vi "RT Main_V1 bis.vi"   [LabVIEW 2015]
doc: "This template is for the Queued Message Handler design pattern.\n\nThe Event Handling Loop generates messages based on user interface actions.\n\nThe Message Handling Loop processes messages generated by the Event Handling Loop, or by other messages. The messages are string values, so new messages can be added easily to the Message Cases case structure in the Message Handling Loop. Each message cluster can also provide an optional value for Message Data, which is a variant that can be converted to whatever message-specific data is required."
uses:
  support/Message Queue/Message Queue.lvlib
  Globals/Global - All RT Loop Stop.vi
  Globals/Global - Configuration Options.vi
  Globals/Global - RT Stream Connections.vi
  Globals/Global - Monitoring Variables.vi
  <vilib>/nisyscfg/nisyscfg.lvlib
types:
  T1 = typedef "Message Queue.lvlib/All Real-Time Message Queues.ctl" = cluster{"Message Handler":refnum<queue>, "Acquisition and Logging":refnum<queue>}
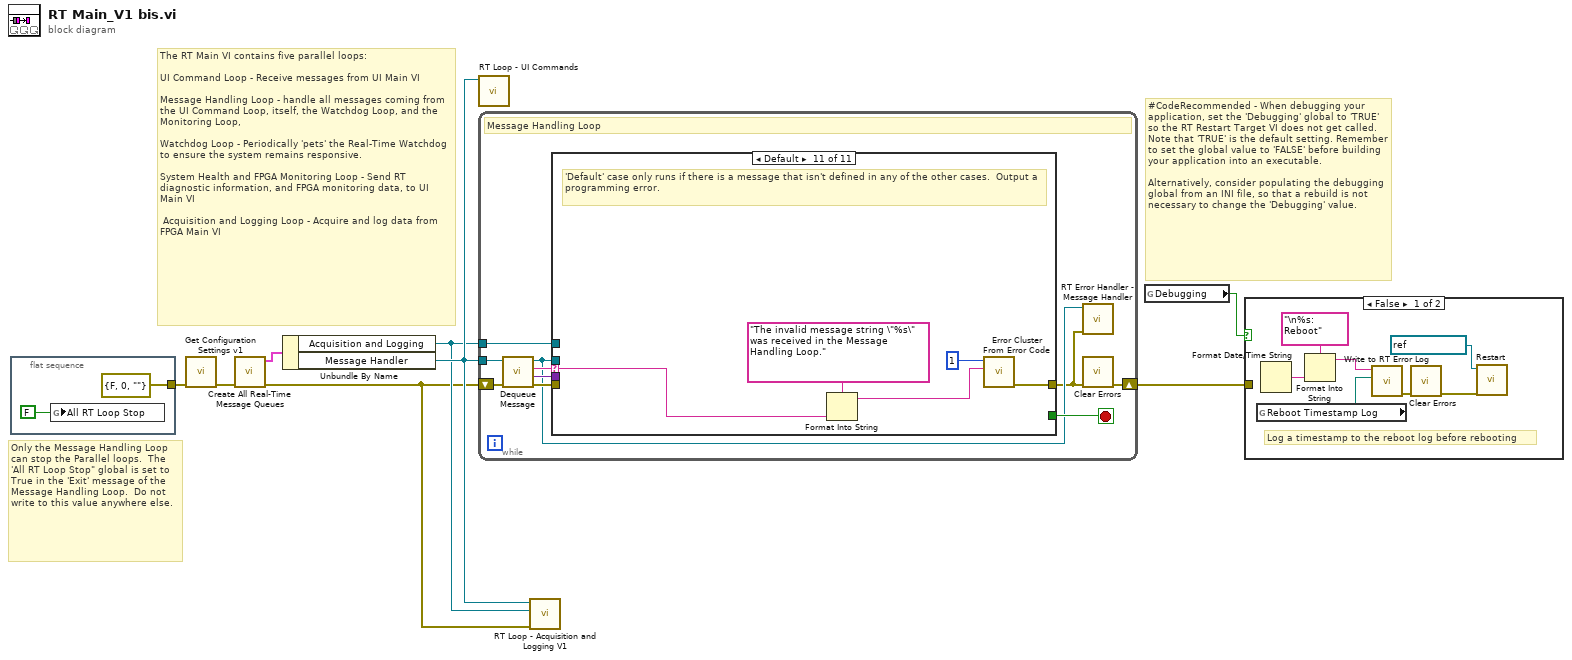
[diagram p0: block diagram]
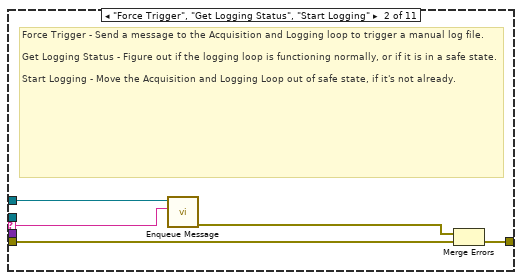
[diagram p4: hidden frame]
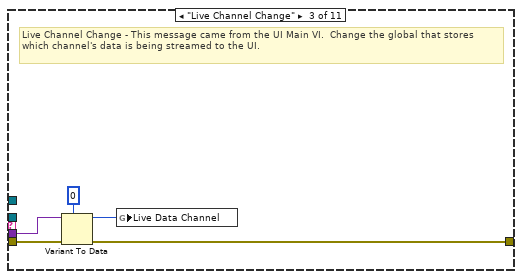
[diagram p5: hidden frame]
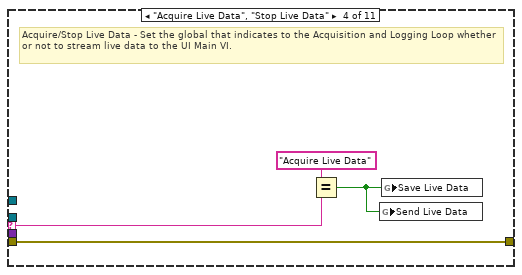
[diagram p6: hidden frame]
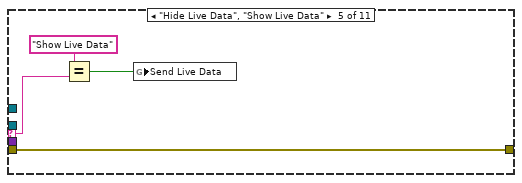
[diagram p7: hidden frame]
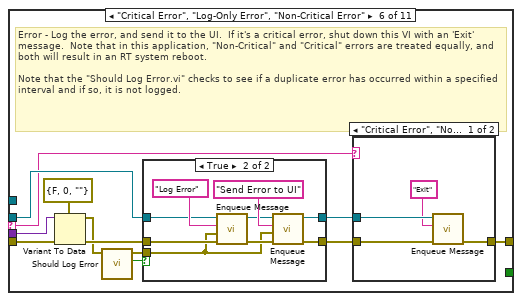
[diagram p8: hidden frame]
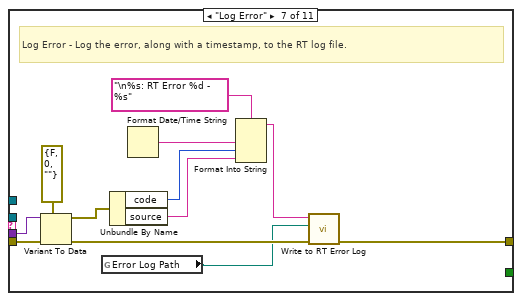
[diagram p11: hidden frame]
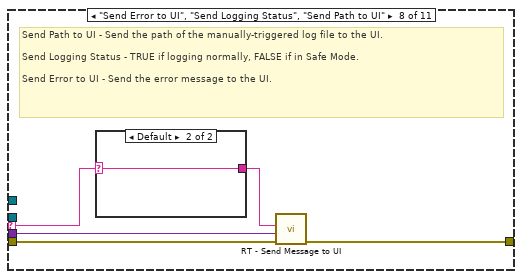
[diagram p12: hidden frame]
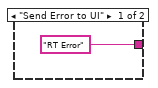
[diagram p13: hidden frame]
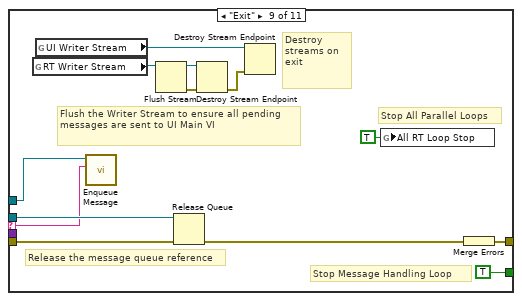
[diagram p14: hidden frame]
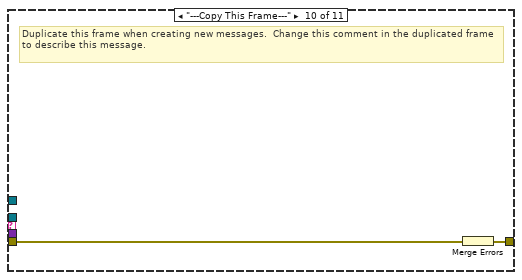
[diagram p15: hidden frame]
diagram:
  # "#CodeRecommended - When debugging your application, set the 'Debugging' global to 'TRUE' so the RT Restart Target VI does not get called.  Note that 'TRUE' is the default setting. Remember to set the global value to 'FALSE' before building your application into an executable.\n\nAlternatively, consider populating the debugging global from an INI file, so that a rebuild is not necessary to change the 'Debugging' value."
  # "The RT Main VI contains five parallel loops:\n\nUI Command Loop - Receive messages from UI Main VI\n\nMessage Handling Loop - handle all messages coming from the UI Command Loop, itself, the Watchdog Loop, and the Monitoring Loop, \n\nWatchdog Loop - Periodically 'pets' the Real-Time Watchdog to ensure the system remains responsive.\n\nSystem Health and FPGA Monitoring Loop - Send RT diagnostic information, and FPGA monitoring data, to UI Main VI\n\n Acquisition and Logging Loop - Acquire and log data from FPGA Main VI"
  # "Only the Message Handling Loop can stop the Parallel loops.  The 'All RT Loop Stop\" global is set to True in the 'Exit' message of the Message Handling Loop.  Do not write to this value anywhere else."
  n1 = flat-sequence {
    tunnel: [errorcluster {"status"=FALSE, "code"=0, "source"=""} ("error constant")] -> w8
    frame #0 {
      n2 = global write "Global - All RT Loop Stop.vi" "All RT Loop Stop"(FALSE) -> ()
    }
  }
  n3 = call "Get Configuration Settings v1.vi"("error in (no error)"=w8) -> ("error out"=w5:errorcluster)  [unwired: 10 in]
  n4 = call "Create All Real-Time Message Queues.vi"("error in (no error)"=w5) -> ("error out"=w1:errorcluster, "Message Queues out"=w4:T1)  [unwired: 9 in]
  n5 = Unbundle By Name(w4) -> ("Acquisition and Logging"=w2:refnum<queue>, "Message Handler"=w3:refnum<queue>)
  n6 = call "RT Loop - UI Commands.vi"("Message Queue"=w3) -> ()  [unwired: 11 in]
  n7 = while {
    tunnel: w3 -> [w15]
    shift-right: [w13] -> w7
    shift-left: w1 -> [w19]
    tunnel: w2 -> [w11]
    stop <- w20 stop-if-true
    # "Message Handling Loop"
    n8 = call "Dequeue Message.vi"("error in (no error)"=w19, "Message Queue"=w15) -> ("error out"=w18:errorcluster, "Message Data"=w16:variant, "Message"=w17:string, "dup Message Queue"=w14:refnum<queue>)  [unwired: 6 in]
    n9 = case "Message Cases" shown="Default" w17 {
      selector: w17 -> [_ w24 _ w34 w36 w45 _ w81 w89 _ w105]
      tunnel: w14 -> [_ _ _ _ _ w46 _ _ w99 _ _]
      tunnel: w18 -> [w21 w26 w31 w35 w39 w48 w79 w84 w95 w101 _]
      tunnel: [w21 w23 w30 w35 w39 w51 w70 w83 w96 w100 w103] -> w12
      tunnel: [_ _ _ _ _ _ _ _ TRUE _ _] -> w20
      tunnel: w16 -> [_ _ w29 _ _ w40 w78 w82 _ _ _]
      tunnel: w11 -> [_ w25 _ _ _ _ _ _ w90 _ _]
      frame "Initialize" {
        # "Initialize - Currently a no-op for the RT Main VI"
      }
      frame "Force Trigger", "Get Logging Status", "Start Logging" {
        # "Force Trigger - Send a message to the Acquisition and Logging loop to trigger a manual log file.\n\nGet Logging Status - Figure out if the logging loop is functioning normally, or if it is in a safe state.\n\nStart Logging - Move the Acquisition and Logging Loop out of safe state, if it's not already."
        n10 = call "Enqueue Message.vi"("Message"=w24, "Message Queue"=w25) -> ("error out"=w22:errorcluster)  [unwired: 8 in, 1 out]
        n11 = Merge Errors(w22, w26) -> (w23:errorcluster)
      }
      frame "Live Channel Change" {
        # "Live Channel Change - This message came from the UI Main VI.  Change the global that stores which channel's data is being streamed to the UI."
        n12 = Variant To Data(error in=w31, type=u32 0, Variant=w29) -> (data=w27:u32, error out=w30:errorcluster)
        n13 = global write "Global - Monitoring Variables.vi" "Live Data Channel"(w27) -> ()
      }
      frame "Acquire Live Data", "Stop Live Data" {
        # "Acquire/Stop Live Data - Set the global that indicates to the Acquisition and Logging Loop whether or not to stream live data to the UI Main VI."
        n14 = Equal?(x="Acquire Live Data", y=w34) -> (x = y?=w32:bool)
        n15 = global write "Global - Monitoring Variables.vi" "Send Live Data"(w32) -> ()
        n16 = global write "Global - Monitoring Variables.vi" "Save Live Data"(w32) -> ()
      }
      frame "Hide Live Data", "Show Live Data" {
        n17 = Equal?(x="Show Live Data", y=w36) -> (x = y?=w37:bool)
        n18 = global write "Global - Monitoring Variables.vi" "Send Live Data"(w37) -> ()
      }
      frame "Critical Error", "Log-Only Error", "Non-Critical Error" {
        # "Error - Log the error, and send it to the UI.  If it's a critical error, shut down this VI with an 'Exit' message.  Note that in this application, \"Non-Critical\" and \"Critical\" errors are treated equally, and both will result in an RT system reboot.\n\nNote that the \"Should Log Error.vi\" checks to see if a duplicate error has occurred within a specified interval and if so, it is not logged."
        n19 = Variant To Data(error in=w48, type=errorcluster {"status"=FALSE, "code"=0, "source"=""} ("error out"), Variant=w40) -> (data=w43:errorcluster, error out=w49:errorcluster)
        n20 = call "Should Log Error.vi"("error to report"=w43) -> ("Should Log Error?"=w41:bool, "dup error to report"=w42:errorcluster)  [unwired: 9 in]
        n21 = case shown="True" w41 {
          tunnel: [w53 w60] -> w47
          tunnel: [w52 w59] -> w44
          tunnel: w46 -> [w52 w58]
          tunnel: w49 -> [w53 w55]
          tunnel: w42 -> [_ w54]
          frame False {
          }
          frame True {
            n22 = call "Enqueue Message.vi"("error in (no error)"=w55, "Message Data"=w54, "Message"="Log Error", "Message Queue"=w58) -> ("error out"=w56:errorcluster, "dup Message Queue"=w57:refnum<queue>)  [unwired: 6 in]
            n23 = call "Enqueue Message.vi"("error in (no error)"=w56, "Message Data"=w54, "Message"="Send Error to UI", "Message Queue"=w57) -> ("error out"=w60:errorcluster, "dup Message Queue"=w59:refnum<queue>)  [unwired: 6 in]
          }
        }
        n24 = case shown="\"Critical Error\", \"Non-Critical Error\"" w45 {
          tunnel: w47 -> [w66 w67]
          tunnel: w44 -> [w64 _]
          tunnel: [w65 w67] -> w51
          frame "Critical Error", "Non-Critical Error" {
            n25 = call "Enqueue Message.vi"("error in (no error)"=w66, "Message"="Exit", "Message Queue"=w64) -> ("error out"=w65:errorcluster)  [unwired: 7 in, 1 out]
          }
          frame Default {
          }
        }
      }
      frame "Log Error" {
        # "Log Error - Log the error, along with a timestamp, to the RT log file."
        n26 = Variant To Data(error in=w79, type=errorcluster {"status"=FALSE, "code"=0, "source"=""} ("error constant"), Variant=w78) -> (data=w73:errorcluster, error out=w76:errorcluster)
        n27 = global read "Global - Configuration Options.vi" "Error Log Path"() -> (w68:path)
        n28 = Unbundle By Name(w73) -> ("code"=w72:i32, "source"=w71:string)
        n29 = Format Date/Time String() -> (date/time string=w74:string)  [unwired: 3 in]
        n30 = Format Into String(format string="\n%s: RT Error %d - %s", w74, w72, w71) -> (resulting string=w69:string)  [unwired: 2 in, 1 out]
        n31 = call "Write to RT Error Log.vi"("error in (no error)"=w76, "Error Log Path"=w68, "Log Entry"=w69) -> ("error out"=w70:errorcluster)  [unwired: 8 in]
      }
      frame "Send Error to UI", "Send Logging Status", "Send Path to UI" {
        # "Send Path to UI - Send the path of the manually-triggered log file to the UI.\n\nSend Logging Status - TRUE if logging normally, FALSE if in Safe Mode.\n\nSend Error to UI - Send the error message to the UI."
        n32 = case shown="Default" w81 {
          selector: w81 -> [_ w86]
          tunnel: ["RT Error" ("Message") w86] -> w80
          frame "Send Error to UI" {
          }
          frame Default {
          }
        }
        n33 = call "RT - Send Message to UI.vi"("error in (no error)"=w84, "Message Data"=w82, "Message"=w80) -> ("error out"=w83:errorcluster)  [unwired: 8 in]
      }
      frame "Exit" {
        # "Flush the Writer Stream to ensure all pending messages are sent to UI Main VI"
        # "Destroy streams on exit"
        # "Stop Message Handling Loop"
        # "Stop All Parallel Loops"
        # "Release the message queue reference"
        n34 = global read "Global - RT Stream Connections.vi" "RT Writer Stream"() -> (w93:refnum<k21>)
        n35 = global read "Global - RT Stream Connections.vi" "UI Writer Stream"() -> (w92:refnum<k21>)
        n36 = call "Enqueue Message.vi"("Message"=w89, "Message Queue"=w90) -> ()  [unwired: 8 in, 2 out]
        n37 = Flush Stream(11:w93) -> (0:w87:errorcluster, 3:w88:refnum<k21>)  [unwired: 3 in, 1 out]
        n38 = Release Queue(queue=w99, error in (no error)=w95) -> (error out=w97:errorcluster)  [unwired: 1 in, 2 out]
        n39 = Destroy Stream Endpoint(8:w87, 11:w88) -> (0:w91:errorcluster)
        n40 = Destroy Stream Endpoint(8:w91, 11:w92) -> ()  [unwired: 1 out]
        n41 = global write "Global - All RT Loop Stop.vi" "All RT Loop Stop"(TRUE ("Stop Monitoring Loops")) -> ()
        n42 = Merge Errors(w97) -> (w96:errorcluster)
      }
      frame "---Copy This Frame---" {
        # "Duplicate this frame when creating new messages.  Change this comment in the duplicated frame to describe this message."
        n43 = Merge Errors(w101) -> (w100:errorcluster)
      }
      frame Default {
        # "'Default' case only runs if there is a message that isn't defined in any of the other cases.  Output a programming error."
        n44 = Format Into String(format string="The invalid message string \"%s\" was received in the Message Handling Loop." ("Unknown Message Error Text"), w105) -> (resulting string=w102:string)  [unwired: 2 in, 1 out]
        n45 = call <vilib>:"Error Cluster From Error Code.vi"("error message (\"\")"=w102, "error code (0)"=1) -> ("error out"=w103:errorcluster)  [unwired: 7 in]
      }
    }
    n46 = call "RT Error Handler - Message Handler.vi"("error in (no error)"=w12, "Message Queue"=w14) -> ()  [unwired: 9 in, 1 out]
    n47 = call <vilib>:"Clear Errors.vi"("error in (no error)"=w12) -> ("error out"=w13:errorcluster)  [unwired: 5 in, 1 out]
  }
  n48 = call "RT Loop - Acquisition and Logging V1.vi"("error in (no error)"=w1, "Acquisition and Logging Queue"=w2, "Message Queue"=w3) -> ()  [unwired: 9 in]
  n49 = global read "Global - Configuration Options.vi" "Debugging"() -> (w6:bool)
  n50 = case shown="False" w6 {
    tunnel: w7 -> [_ _]
    frame False {
      # "Log a timestamp to the reboot log before rebooting"
      n51 = global read "Global - Configuration Options.vi" "Reboot Timestamp Log"() -> (w109:path)
      n52 = Format Date/Time String() -> (date/time string=w111:string)  [unwired: 3 in]
      n53 = Format Into String(format string="\n%s: Reboot", w111) -> (resulting string=w110:string)  [unwired: 2 in, 1 out]
      n54 = call "Write to RT Error Log.vi"("Error Log Path"=w109, "Log Entry"=w110) -> ("error out"=w113:errorcluster)  [unwired: 9 in]
      n55 = call <vilib>:"Clear Errors.vi"("error in (no error)"=w113) -> ("error out"=w108:errorcluster)  [unwired: 5 in, 1 out]
      n56 = call <vilib>:"Restart.vi"("error in (no error)"=w108, "Session in"=refnum<k21> "localhost" ("session in")) -> ()  [unwired: 7 in, 3 out]
    }
    frame True {
    }
  }
